vi "Accept TLS for other TCP.vi"(8 "error in (no error)":errorcluster, 10 "TCP Connection In":refnum<k5>, 11 "Websocket Server in":refnum<class "Websocket Server.lvclass">) -> (0 "error out":errorcluster, 2 "TCP Connection":refnum<k5>, 3 "Websocket Server out":refnum<class "Websocket Server.lvclass">)   [LabVIEW 2020, in "Stream-Websocket.lvlib" / "Websocket Server.lvclass"]
doc: "This VI allows using the TLS configuration for this WebSocket server to perform the TLS handshake on an external TCP reference. This can be useful when running another TCP connection as a server that can be covered by the same certificate as is used with the WebSocket server."
uses:
  Websocket Server.lvclass
  Websocket Server.lvclass/Websocket Server.ctl
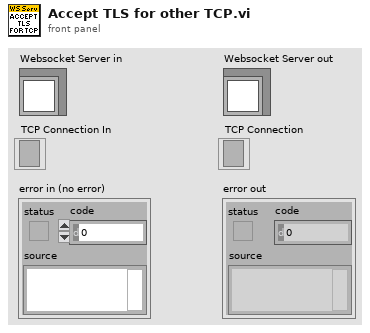
[diagram p1: front panel]
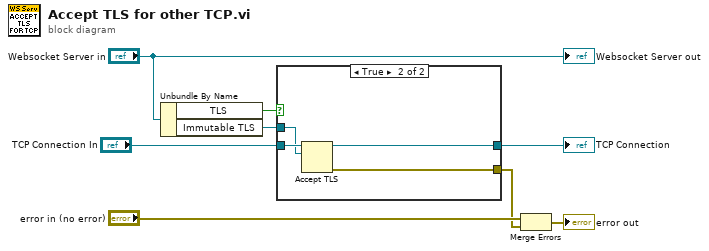
[diagram p0: block diagram]
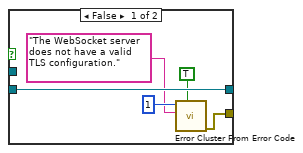
[diagram p2: hidden frame]
diagram:
  n1 = Unbundle By Name("Websocket Server in") -> ("TLS"=w6:bool, "Immutable TLS"=w5:refnum<k36>)
  n2 = case shown="True" w6 {
    tunnel: w5 -> [_ w15]
    tunnel: "TCP Connection In" -> [w13 w17]
    tunnel: [w13 w16] -> w3
    tunnel: [w12 w14] -> w1
    frame False {
      n3 = call <vilib>:"Error Cluster From Error Code.vi"("show call chain? (False)"=TRUE, "error message (\"\")"="The WebSocket server does not have a valid TLS configuration.", "error code (0)"=1) -> ("error out"=w12:errorcluster)  [unwired: 6 in]
    }
    frame True {
      n4 = Accept TLS(10:w15, 11:w17) -> (0:w14:errorcluster, 3:w16:refnum<k5>)  [unwired: 2 in, 1 out]
    }
  }
  "TCP Connection" <- w3
  n5 = Merge Errors("error in (no error)", w1) -> (→"error out":errorcluster)
  "Websocket Server out" <- "Websocket Server in"
